vi "XiXi-1.vi"(7 "VI路径":path, 10 "X[-1]":dbl, 11 "Xi":dbl[](array[numeric])) -> (3 "Yi":dbl[](array[numeric]))   [LabVIEW 2012]
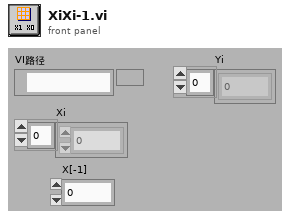
[diagram p1: front panel]
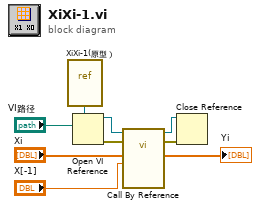
[diagram p0: block diagram]
diagram:
  n1 = vi-ref "XiXi-1(原型）.vi"() -> (w9:refnum<vi>)
  n2 = Open VI Reference(type specifier VI Refnum (for type only)=w9, vi path="VI路径") -> (vi reference=w8:refnum<vi>, error out=w5:errorcluster)  [unwired: 4 in]
  n3 = call-by-ref "?"(reference=w8, error in=w5, "X[-1]"="X[-1]", "Xi"="Xi") -> (reference out=w7:refnum<vi>, error out=w6:errorcluster, "Yi"=→"Yi":dbl[])  [unwired: 9 in]
  n4 = Close Reference(reference=w7, error in (no error)=w6) -> ()  [unwired: 1 out]
